vi "myBOT_Nonlinearities.vi"(10 "Nonlinear Behavior?":bool, 11 "Tmot_in":dbl) -> (3 "Tmot_out":dbl)   [LabVIEW 2013]
doc: "This VI simulates Non-Linear Behavior. Created for the myRIO Balancing Robot Project. See https://decibel.ni.com/content/groups/myrio-balancing-robot for more information and example projects."
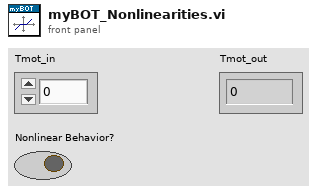
[diagram p1: front panel]
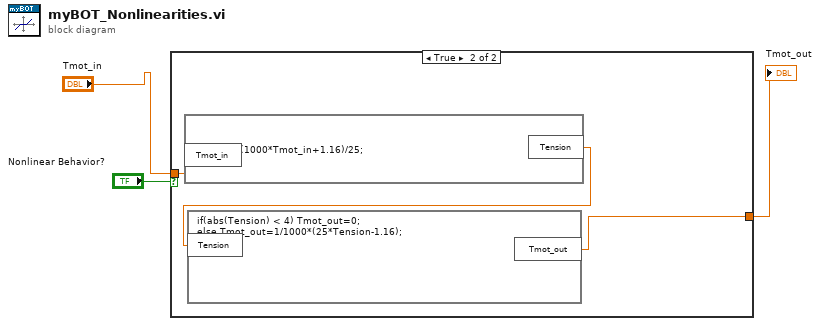
[diagram p0: block diagram]
diagram:
  n1 = case shown="True" "Nonlinear Behavior?" {
    tunnel: "Tmot_in" -> [w4 w7]
    tunnel: [w4 w5] -> w2
    frame False {
    }
    frame True {
      n2 = formula code="Tension=(1000*Tmot_in+1.16)/25;" ("Formula Node 2")("Tmot_in"=w7) -> ("Tension"=w6:dbl)
      n3 = formula code="if(abs(Tension) < 4) Tmot_out=0;\nelse Tmot_out=1/1000*(25*Tension-1.16);" ("Formula Node 3")("Tension"=w6) -> ("Tmot_out"=w5:dbl)
    }
  }
  "Tmot_out" <- w2
